vi "writeSGL.vi"(8 "error in (no error)":errorcluster, 10 "Input":sgl, 11 "ModbusBuffer in":refnum<class "ModbusBufferBuilder.lvclass">) -> (0 "error out":errorcluster, 3 "ModbusBuffer out":refnum<class "ModbusBufferBuilder.lvclass">)   [LabVIEW 2016, in "ModbusBufferBuilder.lvclass"]
uses:
  ModbusBufferBuilder.lvclass
  ModbusBufferBuilder.lvclass/ModbusBufferBuilder.ctl
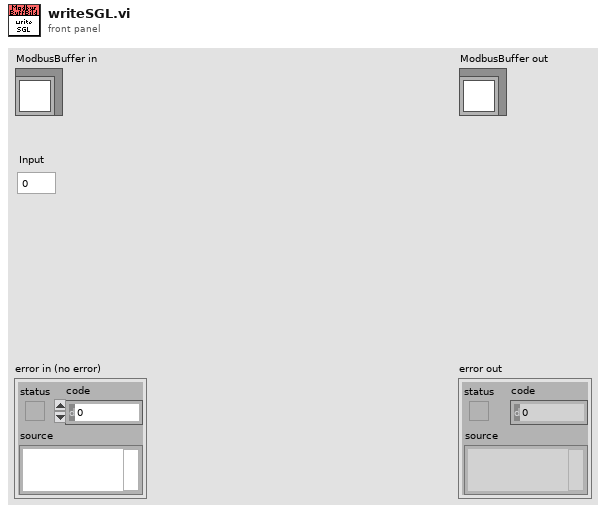
[diagram p1: front panel]
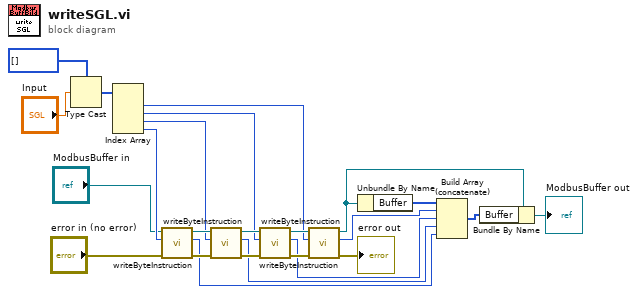
[diagram p0: block diagram]
diagram:
  n1 = Type Cast(type=u8[] [], x="Input") -> (*(type *) &x=w13:u8[])
  n2 = Index Array(array=w13) -> (element #1=w12:u8, element #2=w11:u8, element #3=w10:u8, element #4=w9:u8)  [unwired: 4 in]
  n3 = call "writeByteInstruction.vi"("error in (no error)"="error in (no error)", "Input"=w9, "ModbusBuffer in"="ModbusBuffer in") -> ("error out"=w19:errorcluster, "Output"=w2:u16, "ModbusBuffer out"=w23:refnum<class "ModbusBufferBuilder.lvclass">)  [unwired: 6 in]
  n4 = call "writeByteInstruction.vi"("error in (no error)"=w19, "Input"=w10, "ModbusBuffer in"=w23) -> ("error out"=w18:errorcluster, "Output"=w3:u16, "ModbusBuffer out"=w22:refnum<class "ModbusBufferBuilder.lvclass">)  [unwired: 6 in]
  n5 = call "writeByteInstruction.vi"("error in (no error)"=w18, "Input"=w11, "ModbusBuffer in"=w22) -> ("error out"=w17:errorcluster, "Output"=w4:u16, "ModbusBuffer out"=w21:refnum<class "ModbusBufferBuilder.lvclass">)  [unwired: 6 in]
  n6 = call "writeByteInstruction.vi"("error in (no error)"=w17, "Input"=w12, "ModbusBuffer in"=w21) -> ("error out"=→"error out":errorcluster, "Output"=w5:u16, "ModbusBuffer out"=w20:refnum<class "ModbusBufferBuilder.lvclass">)  [unwired: 6 in]
  n7 = Unbundle By Name(w20) -> ("Buffer"=w6:u16[])
  n8 = Build Array (concatenate)(w6, w5, w4, w3, w2) -> (w1:u16[])
  n9 = Bundle By Name(cluster=w20, "Buffer"=w1) -> (→"ModbusBuffer out":refnum<class "ModbusBufferBuilder.lvclass">)
